vi "Large File - Simple Example.vi"() -> ()   [LabVIEW 2020]
uses:
  <userlib>/_OpenG.lib/largefile/largefile.llb/LF Write File (STR)__ogtk.vi
  <userlib>/_OpenG.lib/largefile/largefile.llb/LF Read File (STR)__ogtk.vi
panel:
  out "offset out 2":dbl format="%.2f"
  out "eof":dbl format="%.2f"
  out "offset out":dbl format="%.2f"
  out "String":string
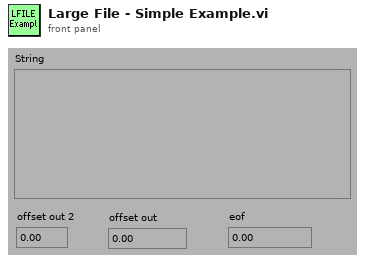
[diagram p1: front panel]
types:
  T1 = enum16{"open", "replace", "create", "open or create", "replace or create", "replace or create with confirmation"}
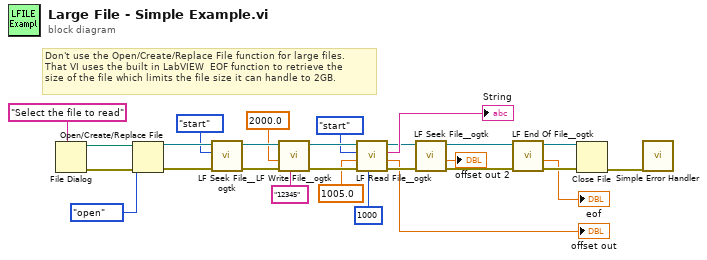
[diagram p0: block diagram]
diagram:
  # "Don't use the Open/Create/Replace File function for large files.\nThat VI uses the built in LabVIEW  EOF function to retrieve the\nsize of the file which limits the file size it can handle to 2GB."
  n1 = File Dialog(7:"Select the file to read" ("prompt")) -> (0:w1:errorcluster, 3:w14:path)  [unwired: 6 in, 2 out]
  n2 = Open/Create/Replace File(file path (use dialog)=w14, error in=w1, operation (0:open)=T1."open") -> (refnum out=w18:refnum<file>, error out=w19:errorcluster)  [unwired: 3 in, 1 out]
  n3 = call <userlib>:"LF Seek File__ogtk.vi"("error in (no error)"=w19, "pos mode (current)"=enum16{"start", "end", "current"}."start", "refnum"=w18) -> ("error out"=w16:errorcluster, "refnum out"=w17:refnum<file>)  [unwired: 2 in, 1 out]
  n4 = call-poly <userlib>:"LF Write File__ogtk.vi"("data"="12345", "error in (no error)"=w16, "offset in (0)"=2000.0, "refnum"=w17) -> ("error out"=w23:errorcluster, "refnum out"=w24:refnum<file>)  [unwired: 4 in, 1 out]
  n5 = call-poly <userlib>:"LF Read File__ogtk.vi"("bytes to read"=1000, "error in (no error)"=w23, "offset in (0)"=1005.0 ("offset in"), "pos mode (current)"=enum16{"start", "end", "current"}."start", "refnum"=w24) -> ("error out"=w12:errorcluster, "offset out"=→"offset out":dbl, "String"=→"String":string, "refnum out"=w11:refnum<file>)  [unwired: 3 in]
  n6 = call <userlib>:"LF Seek File__ogtk.vi"("error in (no error)"=w12, "refnum"=w11) -> ("error out"=w9:errorcluster, "offset out"=→"offset out 2":dbl, "refnum out"=w10:refnum<file>)  [unwired: 3 in]
  n7 = call <userlib>:"LF End Of File__ogtk.vi"("error in (no error)"=w9, "refnum"=w10) -> ("error out"=w22:errorcluster, "offset out"=→"eof":dbl, "refnum out"=w21:refnum<file>)  [unwired: 3 in]
  n8 = Close File(refnum=w21, error in=w22) -> (error out=w25:errorcluster)  [unwired: 1 out]
  n9 = call <vilib>:"Simple Error Handler.vi"("error in (no error)"=w25) -> ()  [unwired: 4 in, 5 out]
